vi "Step-By-Step Tab Window CtrlLogic.vi"(7 "VI Ref (calling VI)":refnum<vi>, 8 "error in (no error)":errorcluster, 11 "CtrlRef":T1) -> ()   [LabVIEW 2017]
doc: "Control logic for a step-by-step tab window. It drives the tab control from the Prev, Next and Finish button references so the user moves through the tabs in order."
uses:
  f6a352cb-c912-43b1-a35d-681ab8cb10a3.vi
panel:
  # "Connector Pane"
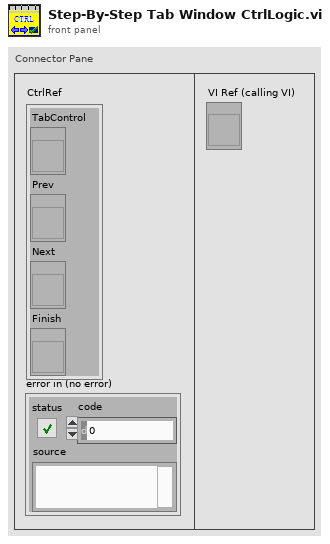
[diagram p1: front panel]
types:
  T1 = cluster{"TabControl":refnum<vi>, "Prev":refnum<vi>, "Next":refnum<vi>, "Finish":refnum<vi>}
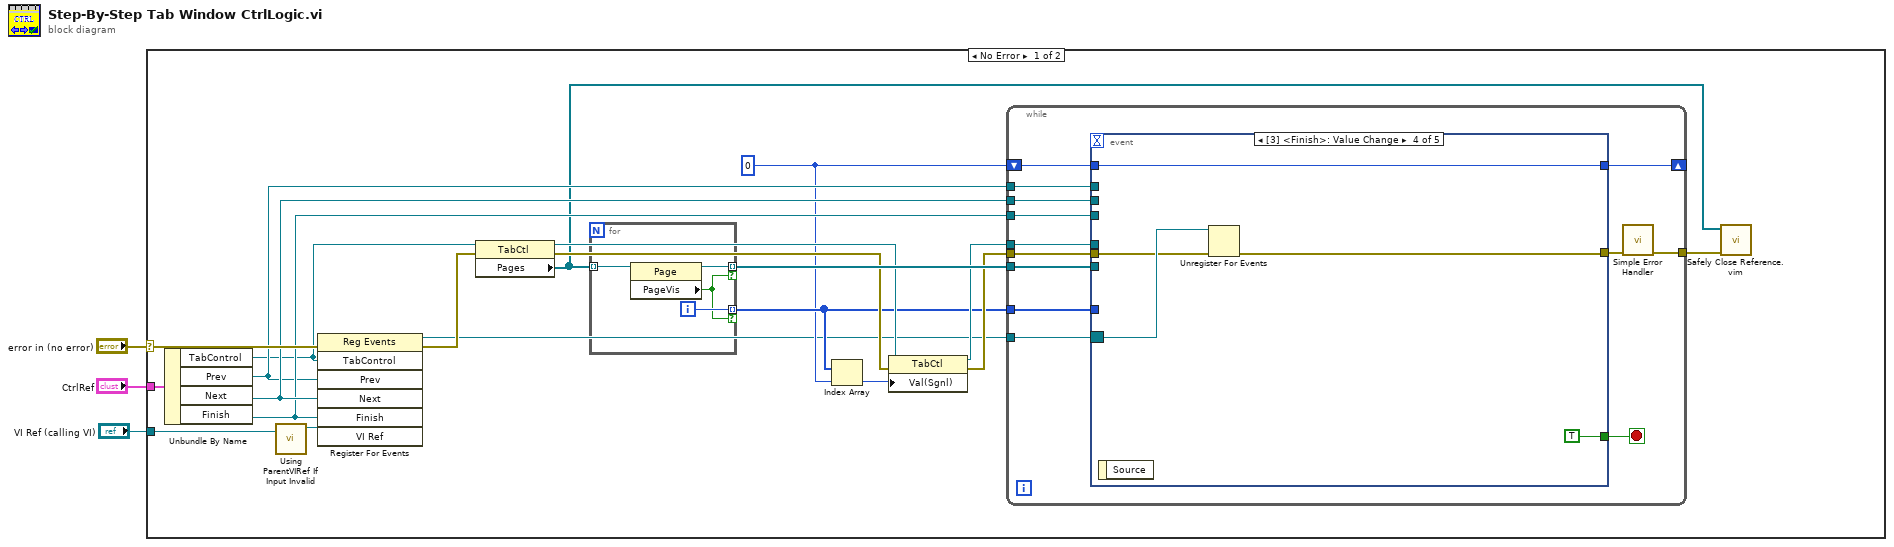
[diagram p0: block diagram]
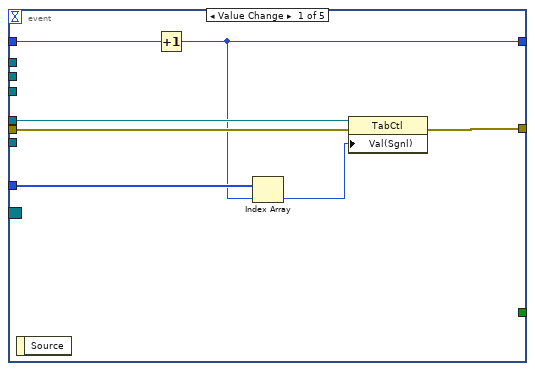
[diagram p2: hidden frame]
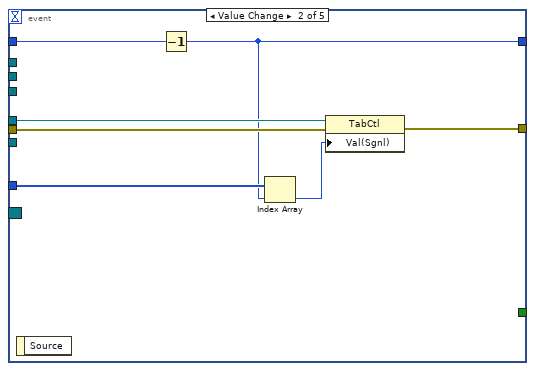
[diagram p3: hidden frame]
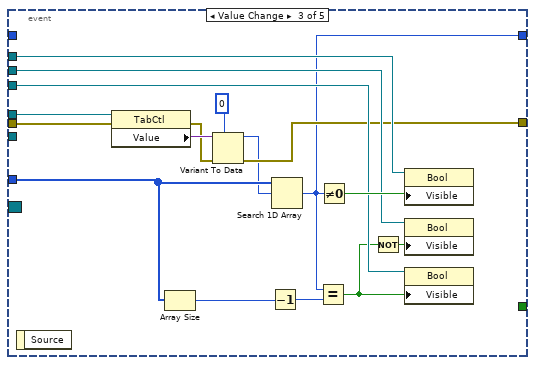
[diagram p4: hidden frame]
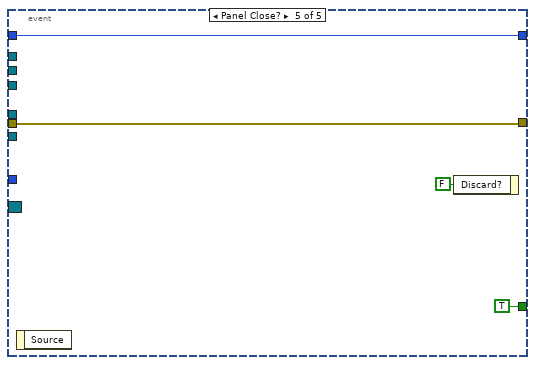
[diagram p5: hidden frame]
diagram:
  n1 = case shown="No Error" "error in (no error)" {
    selector: "error in (no error)" -> [w23 _]
    tunnel: "CtrlRef" -> [w21 _]
    tunnel: "VI Ref (calling VI)" -> [w16 _]
    frame No Error {
      w8 = 0
      n2 = Unbundle By Name(w21) -> ("TabControl"=w15:refnum<vi>, "Prev"=w18:refnum<vi>, "Next"=w20:refnum<vi>, "Finish"=w19:refnum<vi>)
      n3 = call "Using ParentVIRef If Input Invalid.vi"("VI Ref (calling VI)"=w16) -> ("VI Ref"=w17:refnum<vi>)  [unwired: 5 in, 1 out]
      n4 = register-events(error in=w23, w15, w18, w20, w19, w17) -> (reference out=w5:refnum<event-registration>, error out=w22:errorcluster)  [unwired: 1 in]
      n5 = property on="Property Node" class="TabCtl"(reference=w15, error in=w22) -> (reference out=w11:refnum<vi>, error out=w13:errorcluster, "Pages"=w6:refnum<vi>[])
      n6 = for {
        tunnel: w6 -> [w27] mode=indexing
        tunnel: [w26] -> w14 mode=indexing if=w24
        tunnel: [w25] -> w9 mode=indexing if=w24
        i -> [w25]
        n7 = property on="Property Node" class="Page"(reference=w27) -> (reference out=w26:refnum<vi>, "PageVis"=w24:bool)  [unwired: 1 in, 1 out]
      }
      n8 = Index Array(array=w9, index=w8) -> (element=w7:i32)
      n9 = property on="Property Node" class="TabCtl"(reference=w11, error in=w13, "Val(Sgnl)"=w7) -> (reference out=w10:refnum<vi>, error out=w12:errorcluster)
      n10 = while {
        tunnel: w5 -> [w40]
        tunnel: w10 -> [w39]
        tunnel: w12 -> [w38]
        tunnel: w18 -> [w36]
        tunnel: w20 -> [w35]
        tunnel: w19 -> [w34]
        tunnel: [w32] -> w4
        tunnel: w14 -> [w31]
        tunnel: w9 -> [w30]
        shift-right: [w28] -> _
        shift-left: w8 -> [w29]
        stop <- w37 stop-if-true
        n11 = event shown="[3] <Finish>: Value Change" {
          selector: w40 -> [_ _ _ w74 _]
          dyn-events: _ -> [_ _ _ _ _]
          timeout: _ -> [_ _ _ _ _]
          tunnel: w39 -> [w47 w54 w70 _ _]
          tunnel: w38 -> [w44 w53 w71 w73 w77]
          tunnel: [w46 w52 w59 w72 w77] -> w33
          tunnel: [_ _ _ TRUE TRUE] -> w37
          tunnel: w36 -> [_ _ w68 _ _]
          tunnel: w35 -> [_ _ w65 _ _]
          tunnel: w34 -> [_ _ w64 _ _]
          tunnel: w31 -> [_ _ _ _ _]
          tunnel: w30 -> [w43 w50 w57 _ _]
          tunnel: w29 -> [w45 w51 _ w75 w80]
          tunnel: [w42 w49 w55 w75 w80] -> w28
          event Value Change {
            n12 = event-data() -> ()  [unwired: 1 in, 1 out]
            n13 = Increment(x=w45) -> (x+1=w42:i32)
            n14 = Index Array(array=w43, index=w42) -> (element=w41:i32)
            n15 = property class="TabCtl"(reference=w47, error in=w44, "Val(Sgnl)"=w41) -> (error out=w46:errorcluster)  [unwired: 1 out]
          }
          event Value Change {
            n16 = event-data() -> ()  [unwired: 1 in, 1 out]
            n17 = Decrement(x=w51) -> (x-1=w49:i32)
            n18 = Index Array(array=w50, index=w49) -> (element=w48:i32)
            n19 = property class="TabCtl"(reference=w54, error in=w53, "Val(Sgnl)"=w48) -> (error out=w52:errorcluster)  [unwired: 1 out]
          }
          event Value Change {
            n20 = event-data() -> ()  [unwired: 1 in, 1 out]
            n21 = property class="TabCtl"(reference=w70, error in=w71) -> (error out=w60:errorcluster, "Value"=w67:variant)  [unwired: 1 out]
            n22 = Array Size(array=w57) -> (size(s)=w58:i32)
            n23 = Variant To Data(error in=w60, type=0, Variant=w67) -> (data=w56:i32, error out=w59:errorcluster)
            n24 = Decrement(x=w58) -> (x-1=w66:i32)
            n25 = Search 1D Array(1D array=w57, element=w56) -> (index of element=w55:i32)  [unwired: 1 in]
            n26 = Equal?(x=w55, y=w66) -> (x = y?=w63:bool)
            n27 = Not Equal To 0?(x=w55) -> (x != 0?=w69:bool)
            n28 = Not(x=w63) -> (.not. x?=w62:bool)
            n29 = property class="Bool"(reference=w68, "Visible"=w69) -> ()  [unwired: 1 in, 2 out]
            n30 = property class="Bool"(reference=w65, "Visible"=w62) -> ()  [unwired: 1 in, 2 out]
            n31 = property class="Bool"(reference=w64, "Visible"=w63) -> ()  [unwired: 1 in, 2 out]
          }
          event Value Change {
            n32 = event-data() -> ()  [unwired: 1 in, 1 out]
            n33 = Unregister For Events(event registration refnum=w74, error in=w73) -> (error out=w72:errorcluster)
          }
          event Panel Close? {
            n34 = event-data() -> ()  [unwired: 1 in, 1 out]
            n35 = event-data("Discard?"=FALSE) -> ()  [unwired: 1 in, 1 out]
          }
        }
        n36 = call <vilib>:"Simple Error Handler.vi"("error in (no error)"=w33) -> ("error out"=w32:errorcluster)  [unwired: 4 in, 4 out]
      }
      n37 = call "Safely Close Reference.vim"("error in (no error)"=w4, "Reference"=w6) -> ()  [unwired: 9 in, 1 out]
    }
    frame Error {
    }
  }
